vi "SubVI_Integrator.vi"(1 "y_init":dbl, 2 "Init":bool, 3 "T_step [s]":dbl=1.0, 4 "y_min":dbl, 5 "y_max":dbl=inf, 6 "u":dbl) -> (0 "y":dbl)   [LabVIEW 2020]
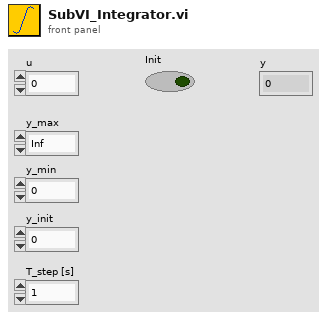
[diagram p1: front panel]
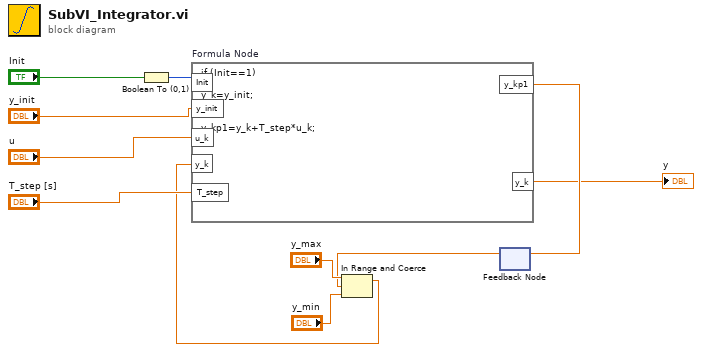
[diagram p0: block diagram]
diagram:
  n1 = Boolean To (0,1)(Boolean="Init") -> (0, 1=w6:i16)
  n2 = feedback #1() -> (w7:dbl)  [unwired: 1 in]
  n3 = In Range and Coerce(upper limit="y_max", x=w7, lower limit="y_min") -> (coerced(x)=w3:dbl)  [unwired: 1 out]
  n4 = formula code="if (Init==1)\n{\ny_k=y_init;\n}\n\ny_kp1=y_k+T_step*u_k;"("u_k"="u", "y_k"=w3, "T_step"="T_step [s]", "Init"=w6, "y_init"="y_init") -> ("y_kp1"=w4:dbl, "y_k"=→"y":dbl)
  n5 = feedback-in #1(w4) -> ()
